vi "DFS Data - Init.vi"() -> (0 "Initial DFS Data":T1)   [LabVIEW 2022 SP3]
doc: "<add documentation here>"
uses:
  DFS Child Node (cluster).ctl
  DFS Node (cluster).ctl
  DFS Data (cluster).ctl
panel:
  # "Development\nControls or indicators that are useful for development or testing, but which are not outputs of the VI."
  # "Input\nInputs to the VI"
  # "Output\nOutputs of the VI"
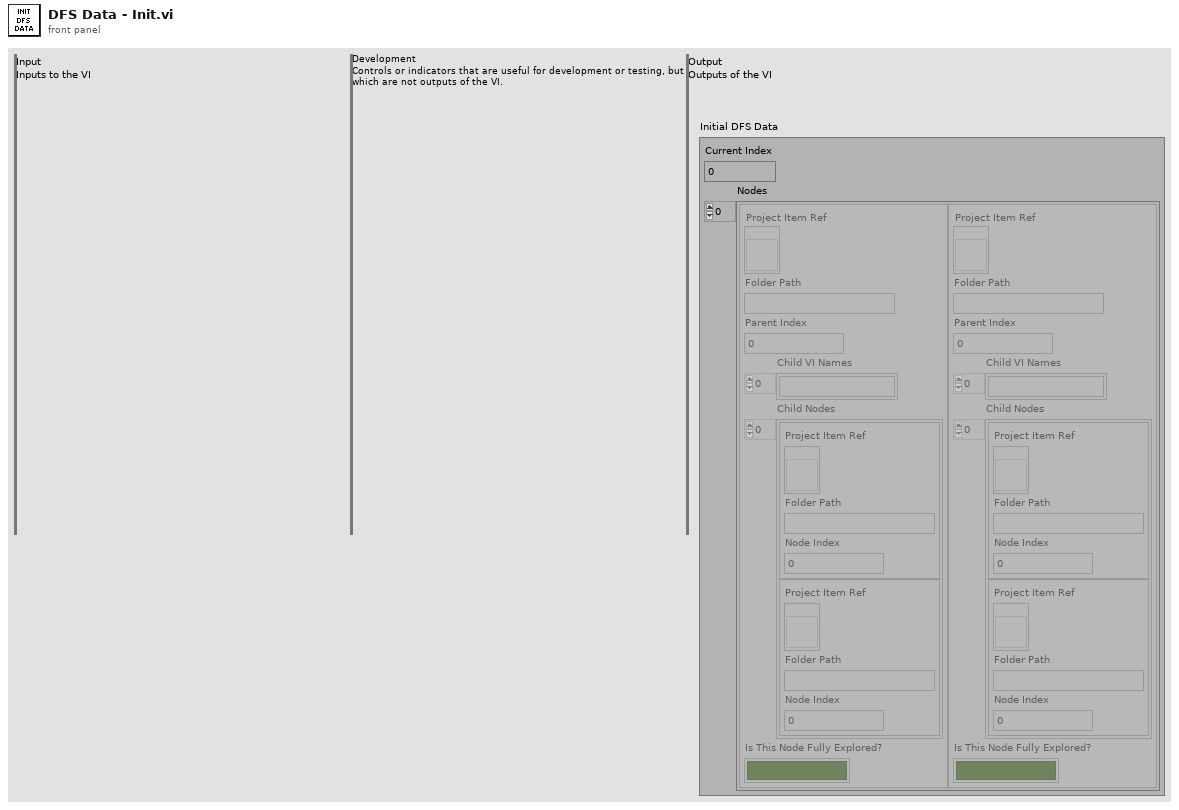
[diagram p1: front panel]
types:
  T1 = typedef "DFS Data (cluster).ctl" = cluster{"Current Index":i32, "Nodes":T2[]}
  T2 = typedef "DFS Node (cluster).ctl" = cluster{"Project Item Ref":refnum<vi>, "Folder Path":string, "Parent Index":i32, "Child VI Names":string[], "Child Nodes":T3[], "Is This Node Fully Explored?":bool}
  T3 = typedef "DFS Child Node (cluster).ctl" = cluster{"Project Item Ref":refnum<vi>, "Folder Path":string, "Node Index":i32}
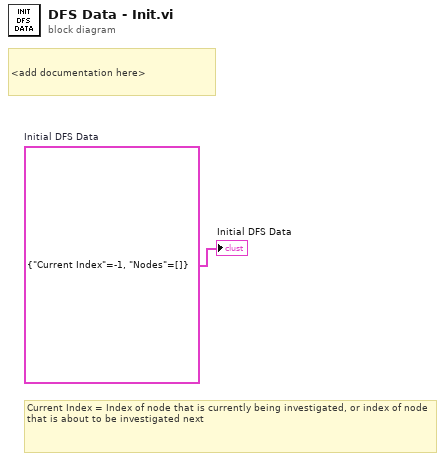
[diagram p0: block diagram]
diagram:
  w1 = T1 {"Current Index"=-1, "Nodes"=[]}  # Initial DFS Data
  # "Current Index = Index of node that is currently being investigated, or index of node that is about to be investigated next"
  # "<add documentation here>"
  "Initial DFS Data" <- w1
